vi "Create (Host Port).vi"(7 "Scheme (None)":string, 10 "Port":u16, 11 "Host":string) -> (3 "URI out":refnum<class "URI.lvclass">)   [LabVIEW 2020, in "URI.lvlib" / "URI.lvclass"]
uses:
  URI.lvclass
  URI.lvclass/URI.ctl
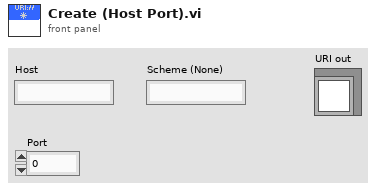
[diagram p1: front panel]
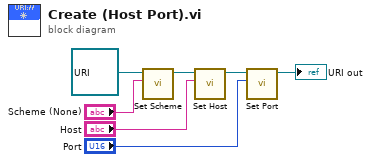
[diagram p0: block diagram]
diagram:
  n1 = call "Set Scheme.vi"("Scheme"="Scheme (None)", "URI in"=refnum<class "URI.lvclass"> refnum) -> ("URI out"=w2:refnum<class "URI.lvclass">)  [unwired: 9 in]
  n2 = call "Set Host.vi"("Host"="Host", "URI in"=w2) -> ("URI out"=w6:refnum<class "URI.lvclass">)  [unwired: 9 in]
  n3 = call "Set Port.vi"("Port"="Port", "URI in"=w6) -> ("URI out"=→"URI out":refnum<class "URI.lvclass">)  [unwired: 9 in]
